vi "FGV_Seek.vi"(8 "Error IN":errorcluster, 9 "Seek (con) IN":u32, 11 "IN or OUT":enum16{"IN", "OUT"}(ring)) -> (0 "Error OUT":errorcluster, 1 "Seek (con) OUT":u32)   [LabVIEW 2017]
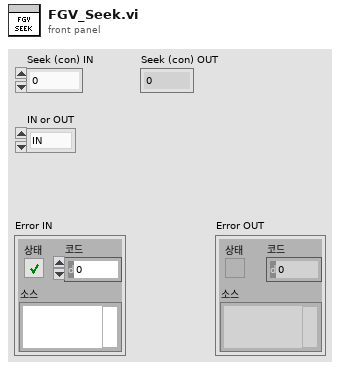
[diagram p1: front panel]
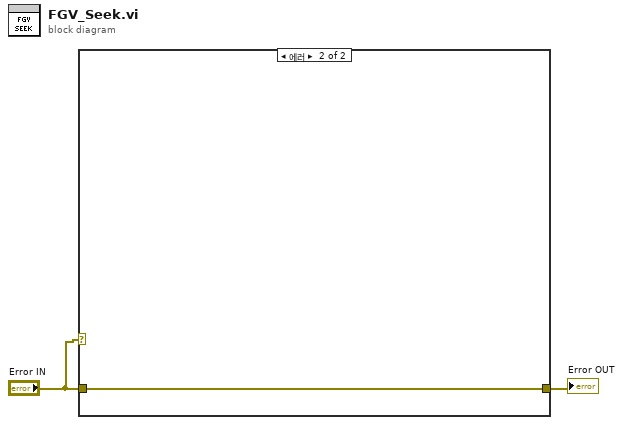
[diagram p0: block diagram]
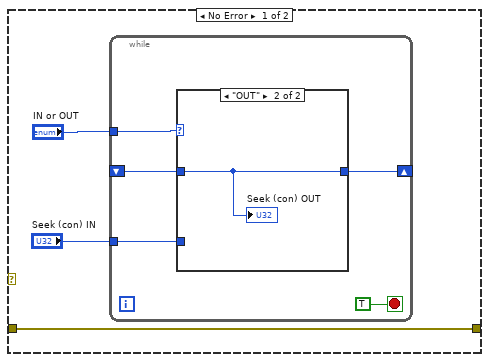
[diagram p2: hidden frame]
diagram:
  n1 = case shown="에러" "Error IN" {
    tunnel: "Error IN" -> [w3 w13]
    tunnel: [w3 w13] -> w1
    frame No Error {
      n2 = while {
        tunnel: "Seek (con) IN" -> [w8]
        shift-right: [w9] -> _
        shift-left: _ -> [w6]
        tunnel: "IN or OUT" -> [w7]
        stop <- TRUE stop-if-true
        n3 = case shown="\"OUT\"" w7 {
          tunnel: [w11 w12] -> w9
          tunnel: w8 -> [w11 _]
          tunnel: w6 -> [_ w12]
          frame "IN", Default {
          }
          frame "OUT" {
            "Seek (con) OUT" <- w12
          }
        }
      }
    }
    frame Error {
    }
  }
  "Error OUT" <- w1
